vi "Find & Convert Attributes.vi"(8 "Error In":errorcluster, 11 "Cluster in":refnum<vi>) -> (0 "Error Out":errorcluster, 2 "Attribute Values":string[](array[string]), 3 "Attribute Names":string[](array[string]))   [LabVIEW 2013, in "JUnit API.lvlib"]
doc: "Converts the attributes cluster provided into an array of attributes and attribute values. Only attributes that have a value (strings with length > 0 and numerics of value >=0) will be output."
uses:
  JUnit API.lvlib
  <vilib>/Utility/VariantDataType/VariantType.lvlib
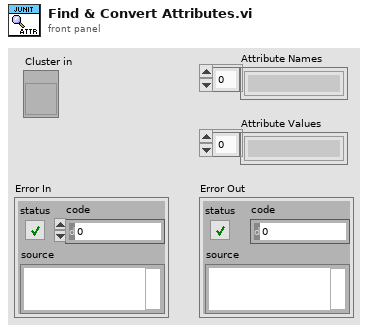
[diagram p1: front panel]
types:
  T1 = typedef "VariantType.lvlib/Type.ctl" = enum8{"Invalid Type", "Void", "I8", "I16", "I32", "I64", "U8", "U16", "U32", "U64", "Single Float", "Double Float", "Extended Float", "Single Complex", "Double Complex", "Extended Complex", "Enum U8", "Enum U16", "Enum U32", "Enum U64", "Single Float With Unit", "Double Float With Unit", "Extended Float With Unit", "Single Complex with Unit", "Double Complex with Unit", "Extended Complex with Unit", "Boolean", "String", "Path", "Picture", "Tag", "Array", "Cluster", "Variant", "LV Variant", "Waveform", "Timestamp", "Digital Waveform", "Digital Data", "ExpressData", "Refnum", "External Data", "VI", "Poly VI", "LabVIEW Class Instance", "Fixed Point"}
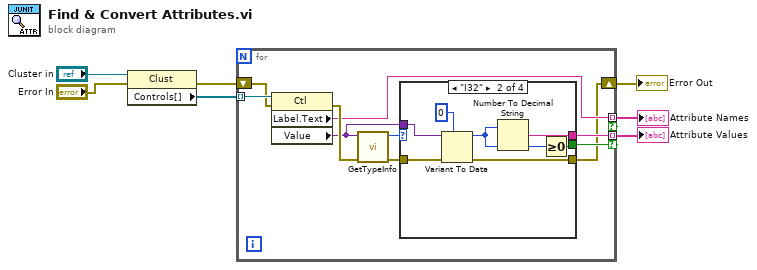
[diagram p0: block diagram]
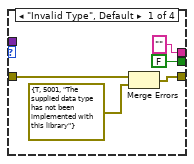
[diagram p2: hidden frame]
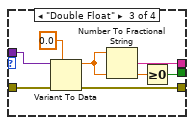
[diagram p3: hidden frame]
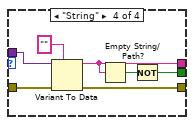
[diagram p4: hidden frame]
diagram:
  n1 = property class="Clust"(reference="Cluster in", error in="Error In") -> (error out=w6:errorcluster, "Controls[]"=w7:refnum<vi>[])  [unwired: 1 out]
  n2 = for {
    tunnel: w7 -> [w17] mode=indexing
    shift-right: [w8] -> w3
    shift-left: w6 -> [w16]
    tunnel: [w11] -> w4 mode=indexing if=w9
    tunnel: [w10] -> w5 mode=indexing if=w9
    n3 = property class="Ctl"(reference=w17, error in=w16) -> (error out=w15:errorcluster, "Label.Text"=w10:string, "Value"=w12:variant)  [unwired: 1 out]
    n4 = call <vilib>:"GetTypeInfo.vi"("error in (no error)"=w15, "Variant"=w12) -> ("error out"=w13:errorcluster, "Type Enum"=w14:T1)  [unwired: 5 in, 3 out]
    n5 = case shown="\"I32\"" w14 {
      tunnel: w13 -> [w22 w28 w35 w43]
      tunnel: [w20 w25 w32 w40] -> w8
      tunnel: w12 -> [_ w29 w36 w42]
      tunnel: ["" w26 w33 w38] -> w11
      tunnel: [FALSE w23 w30 w37] -> w9
      frame "Invalid Type", Default {
        n6 = Merge Errors(w22, errorcluster {"status"=TRUE, "code"=5001, "source"="The supplied data type has not been implemented with this library"} ("error in")) -> (w20:errorcluster)
      }
      frame "I32" {
        n7 = Variant To Data(error in=w28, type=0, Variant=w29) -> (data=w24:i32, error out=w25:errorcluster)
        n8 = Number To Decimal String(number=w24) -> (decimal integer string=w26:string)  [unwired: 1 in]
        n9 = Greater Or Equal To 0?(x=w24) -> (x >= 0?=w23:bool)
      }
      frame "Double Float" {
        n10 = Variant To Data(error in=w35, type=0.0, Variant=w36) -> (data=w31:dbl, error out=w32:errorcluster)
        n11 = Number To Fractional String(number=w31) -> (F-format string=w33:string)  [unwired: 3 in]
        n12 = Greater Or Equal To 0?(x=w31) -> (x >= 0?=w30:bool)
      }
      frame "String" {
        n13 = Variant To Data(error in=w43, type="", Variant=w42) -> (data=w38:string, error out=w40:errorcluster)
        n14 = Empty String/Path?(string/path=w38) -> (empty?=w39:bool)
        n15 = Not(x=w39) -> (.not. x?=w37:bool)
      }
    }
  }
  "Attribute Values" <- w4
  "Attribute Names" <- w5
  "Error Out" <- w3
